vi "Read Sub Panel Coins.vi"(8 "error in (no error)":errorcluster, 11 "Actor_C_MXN in":refnum<class "Actor_C_MXN.lvclass">) -> (0 "error out":errorcluster, 2 "Sub Panel Coins":refnum<vi>, 3 "Actor_C_MXN out":refnum<class "Actor_C_MXN.lvclass">)   [LabVIEW 2019, in "Actor_C_MXN.lvlib" / "Actor_C_MXN.lvclass"]
uses:
  Actor_C_MXN.lvclass
  Actor_C_MXN.lvclass/Actor_C_MXN.ctl
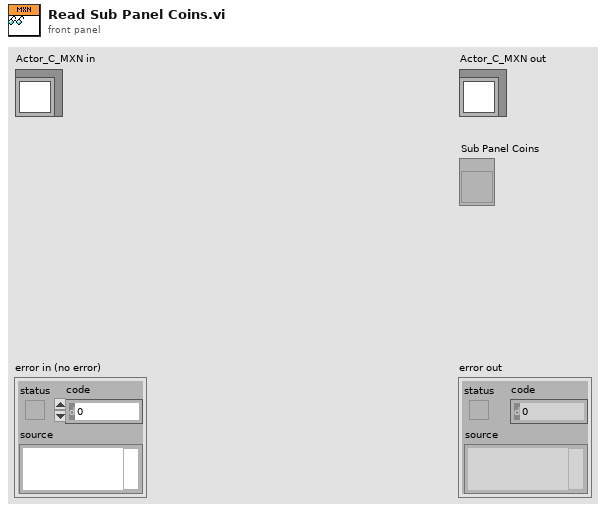
[diagram p1: front panel]
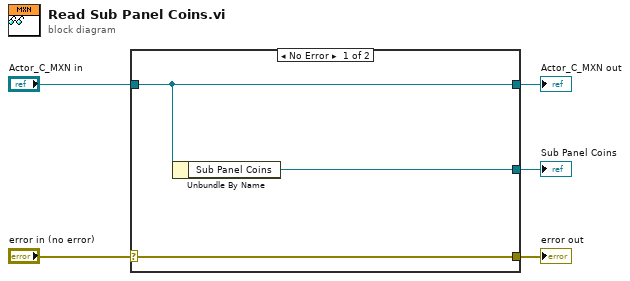
[diagram p0: block diagram]
diagram:
  n1 = case shown="No Error" "error in (no error)" {
    selector: "error in (no error)" -> [w8 w9]
    tunnel: [w8 w9] -> w4
    tunnel: [w7 w10] -> w2
    tunnel: "Actor_C_MXN in" -> [w7 w10]
    tunnel: [w6 _] -> w1
    frame No Error {
      n2 = Unbundle By Name(w7) -> ("Sub Panel Coins"=w6:refnum<vi>)
    }
    frame Error {
    }
  }
  "error out" <- w4
  "Actor_C_MXN out" <- w2
  "Sub Panel Coins" <- w1
